vi "algo.run.HostToFpgaTests.vi"() -> (3 "All Passed?":bool)   [LabVIEW 2020]
panel:
  in  "Filters":string[](array[string])=["hostToFpgaTests", "tests.add", "tests.edit", "tests.remove"]
  in  "error in":errorcluster
  out "error out":errorcluster
  out "Results.out":T1
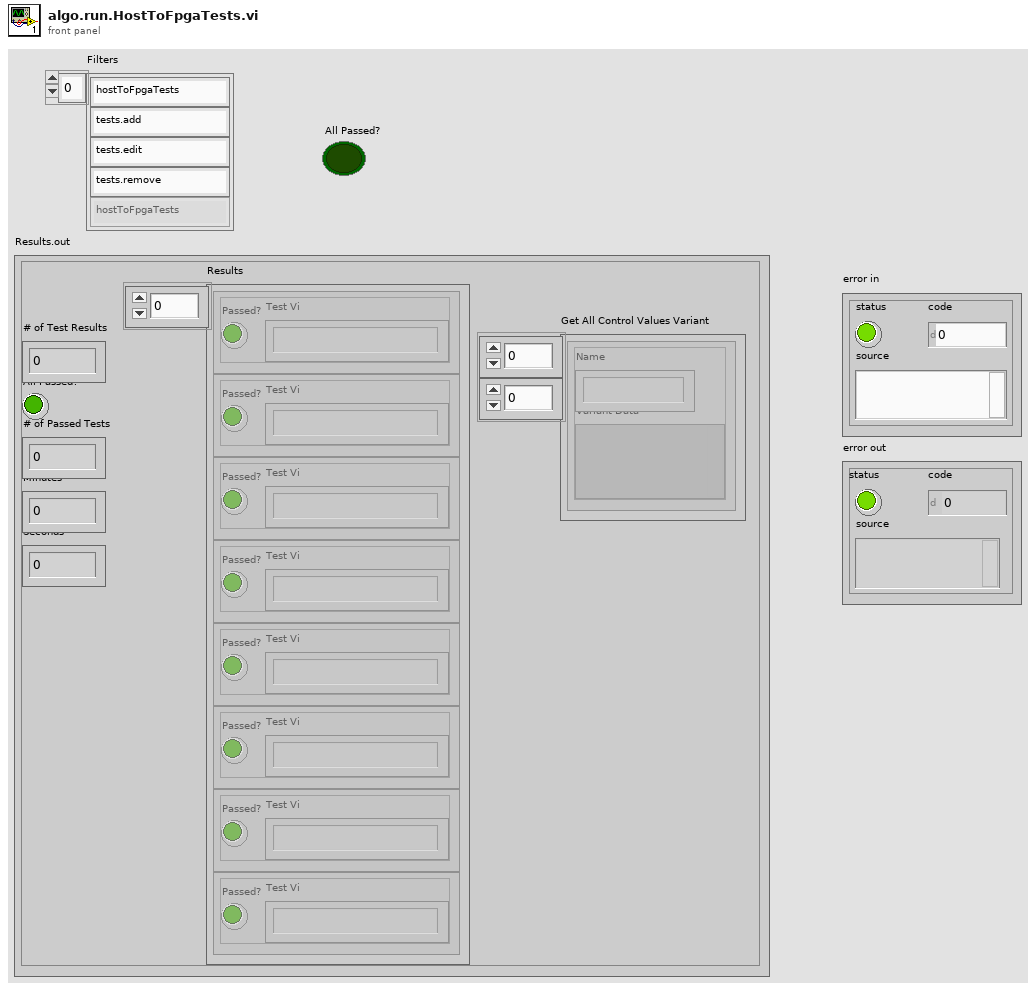
[diagram p1: front panel]
types:
  T1 = cluster{"Results":cluster{"Test Vi":string, "Passed?":bool}[], "# of Test Results":i32, "All Passed?":bool, "# of Passed Tests":i32, "Minutes":u32, "Seconds":u32, "Get All Control Values Variant":cluster{"Name":string, "Variant Data":variant}[][]}
  T2 = cluster{"Filters":string[], "path":path, "error in":errorcluster}
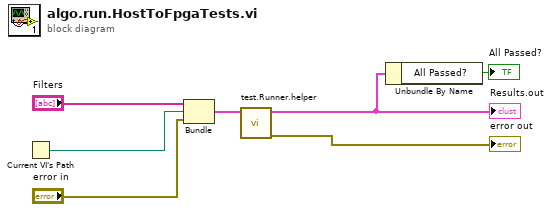
[diagram p0: block diagram]
diagram:
  n1 = Current VI's Path() -> (path=w7:path)
  n2 = Bundle("Filters"="Filters", "path"=w7, "error in"="error in") -> (w6:T2)  [unwired: 1 in]
  n3 = call "test.Runner.helper.vi"("Parameters.in"=w6) -> ("error out"=→"error out":errorcluster, "Results.out"=w1:T1)  [unwired: 9 in]
  "Results.out" <- w1
  n4 = Unbundle By Name(w1) -> ("All Passed?"=→"All Passed?":bool)
